vi "Finish.vi"   [LabVIEW 2015]
doc: "This VI is called just before exiting. It is expected to close I/O refnum, save collected data, etc."
uses:
  <vilib>/Rock Robotics/WPI/Utilities/WPI_GetSetVariantRefNum.vi
types:
  T1 = typedef "WPI_MotorControlDeviceRef.ctl" = cluster{"DeviceStatus":errorcluster, "Type":T2, "PWM":cluster{"PWM Channel":T3, "DeadBand":T4}, "CAN":cluster{"Device Number":u8, "Control Mode":T5, "Semaphore":T6, "Max Vout":dbl, "TalonSRX Control Mode":T7}, "Invert":bool}
  T2 = typedef "WPI_MotorControlType.ctl" = enum16{"PWM", "CAN", "CANTalonSRX"}
  T3 = typedef "FPGA_DIOPWMChannel.ctl" = enum8{"PWM 0", "PWM 1", "PWM 2", "PWM 3", "PWM 4", "PWM 5", "PWM 6", "PWM 7", "PWM 8", "PWM 9", "PWM MXP 0", "PWM MXP 1", "PWM MXP 2", "PWM MXP 3", "PWM MXP 4", "PWM MXP 5", "PWM MXP 6", "PWM MXP 7", "PWM MXP 8", "PWM MXP 9", "Invalid"}
  T4 = typedef "WPI_PWMDeadband.ctl" = cluster{"Name":string, "maxPositivePwm":i32, "minPositivePwm":i32, "centerPwm":i32, "maxNegativePwm":i32, "minNegativePwm":i32, "angularRange":u16}
  T5 = typedef "WPI_CANJaguar_ControlMode.ctl" = enum8{"Percent VBus", "Current", "Speed", "Position", "Voltage"}
  T6 = typedef "Semaphore RefNum" = refnum<k1>
  T7 = typedef "WPI_CANTalonSRX_APIControlMode.ctl" = enum8{"Percent VBus", "Speed", "Position", "Slave", "Unchanged / Invalid", "Voltage Compensation", "Current", "Motion Profile"}
  T8 = typedef "WPI_SwitchDevRef.ctl" = cluster{"DevStatus":errorcluster, "DIO Channel":T9, "CntIndex":T10, "Normally Closed":bool}
  T9 = typedef "FPGA_DIOChannel.ctl" = enum8{"DIO 0", "DIO 1", "DIO 2", "DIO 3", "DIO 4", "DIO 5", "DIO 6", "DIO 7", "DIO 8", "DIO 9", "DIO MXP 0", "DIO MXP 1", "DIO MXP 2", "DIO MXP 3", "DIO MXP 4", "DIO MXP 5", "DIO MXP 6", "DIO MXP 7", "DIO MXP 8", "DIO MXP 9", "DIO MXP 10", "DIO MXP 11", "DIO MXP 12", "DIO MXP 13", "DIO MXP 14", "DIO MXP 15", "Invalid"}
  T10 = typedef "FPGA_CounterCtrSystemIndex.ctl" = enum8{"Ctr 0", "Ctr 1", "Ctr 2", "Ctr 3", "Ctr 4", "Ctr 5", "Ctr 6", "Ctr 7", "Invalid"}
  T11 = typedef "WPI_JoystickDevRef.ctl" = cluster{"Device":T12}
  T12 = typedef "WPI_JoystickDeviceEnum.ctl" = enum16{"USB 0", "USB 1", "USB 2", "USB 3", "USB 4", "USB 5"}
  T13 = typedef "WPI_SolenoidDevRef.ctl" = cluster{"DevStatus":errorcluster, "Pneumatics Control Module":u8, "Forward Solenoid Channel":T14, "Reverse Solenoid Channel":T14}
  T14 = typedef "WPI_SolenoidChannel.ctl" = enum8{"Solenoid 0", "Solenoid 1", "Solenoid 2", "Solenoid 3", "Solenoid 4", "Solenoid 5", "Solenoid 6", "Solenoid 7", "Invalid"}
  T15 = typedef "WPI_RelayDevRef.ctl" = cluster{"DevStatus":errorcluster, "Relay Channel":T16, "Relay Direction":T17}
  T16 = typedef "FPGA_DIORelayChannel.ctl" = enum8{"Relay 0", "Relay 1", "Relay 2", "Relay 3", "Invalid"}
  T17 = typedef "WPI_RelayDirection.ctl" = enum16{"Both directions", "Forward only", "Reverse only"}
  T18 = typedef "WPI_CompressorDevRef.ctl" = cluster{"DevStatus":errorcluster, "Pneumatics Control Module":u8}
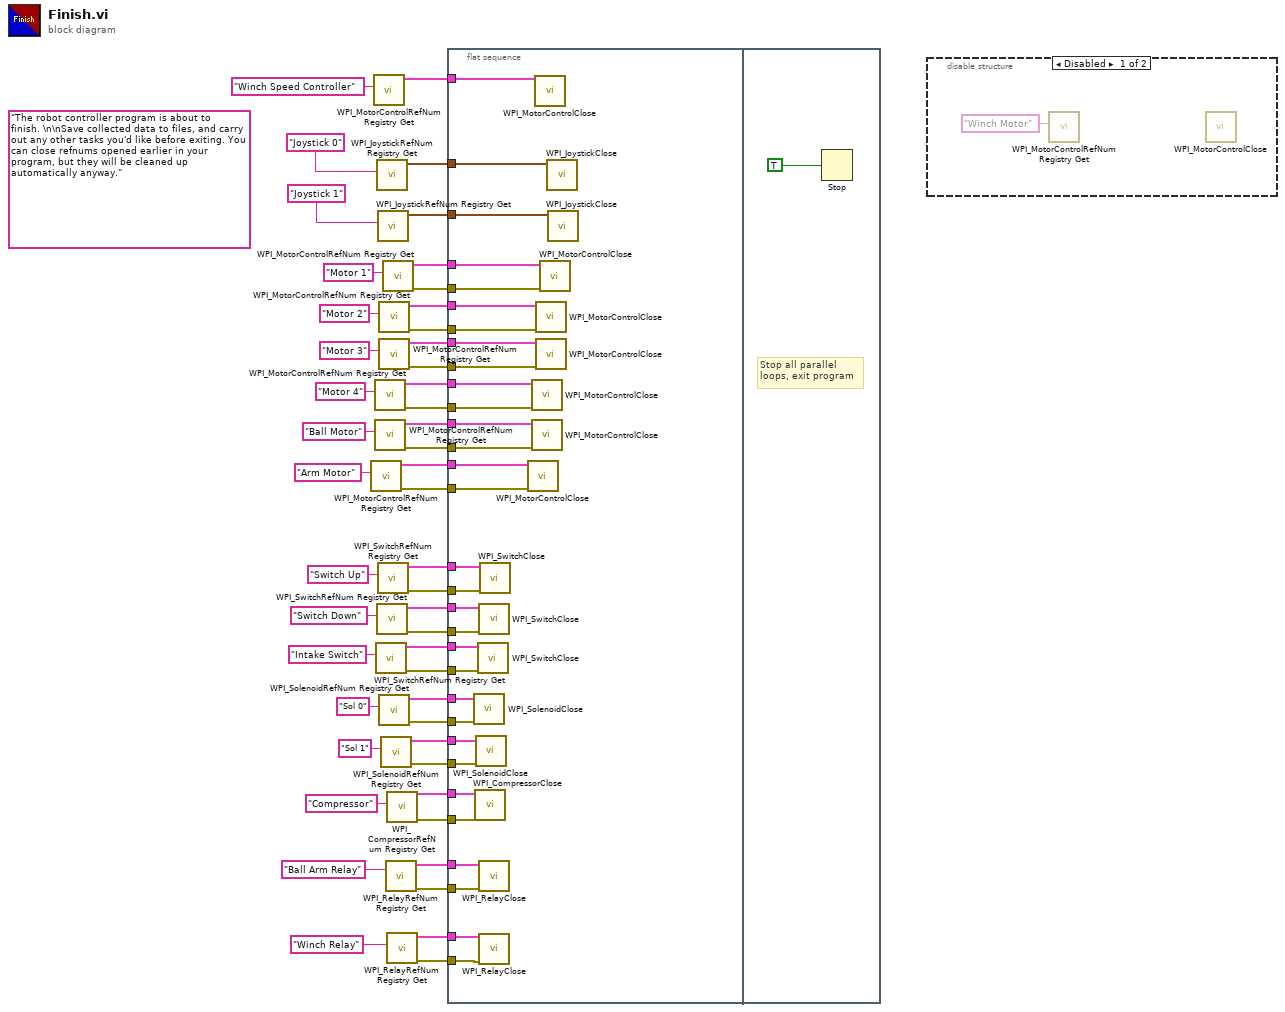
[diagram p0: block diagram]
diagram:
  (unwired) "The robot controller program is about to finish. \n\nSave collected data to files, and carry out any other tasks you'd like before exiting. You can close refnums opened earlier in your program, but they will be cleaned up automatically anyway."
  n1 = call <vilib>:"WPI_MotorControlRefNum Registry Get.vi"("refnum name"="Arm Motor") -> ("error out"=w28:errorcluster, "MotorControlDevRef"=w27:T1)  [unwired: 9 in]
  n2 = call <vilib>:"WPI_MotorControlRefNum Registry Get.vi"("refnum name"="Winch Speed Controller") -> ("MotorControlDevRef"=w2:T1)  [unwired: 9 in, 1 out]
  n3 = call <vilib>:"WPI_MotorControlRefNum Registry Get.vi"("refnum name"="Motor 4") -> ("error out"=w37:errorcluster, "MotorControlDevRef"=w38:T1)  [unwired: 9 in]
  n4 = call <vilib>:"WPI_MotorControlRefNum Registry Get.vi"("refnum name"="Ball Motor") -> ("error out"=w31:errorcluster, "MotorControlDevRef"=w32:T1)  [unwired: 9 in]
  n5 = call <vilib>:"WPI_SwitchRefNum Registry Get.vi"("refnum name"="Intake Switch") -> ("error out"=w19:errorcluster, "SwitchDevRef"=w20:T8)  [unwired: 9 in]
  n6 = call <vilib>:"WPI_JoystickRefNum Registry Get.vi"("refnum name"="Joystick 0") -> ("JoystickDevRef"=w47:T11)  [unwired: 1 in, 9 out]
  n7 = call <vilib>:"WPI_SwitchRefNum Registry Get.vi"("refnum name"="Switch Down") -> ("error out"=w22:errorcluster, "SwitchDevRef"=w21:T8)  [unwired: 9 in]
  n8 = call <vilib>:"WPI_JoystickRefNum Registry Get.vi"("refnum name"="Joystick 1") -> ("JoystickDevRef"=w46:T11)  [unwired: 1 in, 9 out]
  n9 = call <vilib>:"WPI_SwitchRefNum Registry Get.vi"("refnum name"="Switch Up") -> ("error out"=w25:errorcluster, "SwitchDevRef"=w26:T8)  [unwired: 9 in]
  n10 = call <vilib>:"WPI_MotorControlRefNum Registry Get.vi"("refnum name"="Motor 2") -> ("error out"=w40:errorcluster, "MotorControlDevRef"=w39:T1)  [unwired: 9 in]
  n11 = call <vilib>:"WPI_MotorControlRefNum Registry Get.vi"("refnum name"="Motor 3") -> ("error out"=w34:errorcluster, "MotorControlDevRef"=w33:T1)  [unwired: 9 in]
  n12 = call <vilib>:"WPI_SolenoidRefNum Registry Get.vi"("refnum name"="Sol 0") -> ("error out"=w16:errorcluster, "SolenoidDevRef"=w17:T13)  [unwired: 9 in]
  n13 = call <vilib>:"WPI_SolenoidRefNum Registry Get.vi"("refnum name"="Sol 1") -> ("error out"=w13:errorcluster, "SolenoidDevRef"=w12:T13)  [unwired: 9 in]
  n14 = call <vilib>:"WPI_MotorControlRefNum Registry Get.vi"("refnum name"="Motor 1") -> ("error out"=w43:errorcluster, "MotorControlDevRef"=w44:T1)  [unwired: 9 in]
  n15 = call <vilib>:"WPI_RelayRefNum Registry Get.vi"("refnum name"="Ball Arm Relay") -> ("error out"=w5:errorcluster, "RelayDevRef"=w7:T15)  [unwired: 9 in]
  n16 = call <vilib>:"WPI_CompressorRefNum Registry Get.vi"("refnum name"="Compressor") -> ("error out"=w10:errorcluster, "CompressorDevRef"=w11:T18)  [unwired: 9 in]
  n17 = call <vilib>:"WPI_RelayRefNum Registry Get.vi"("refnum name"="Winch Relay") -> ("error out"=w6:errorcluster, "RelayDevRef"=w8:T15)  [unwired: 9 in]
  n18 = flat-sequence {
    tunnel: w47 -> [w79]
    tunnel: w46 -> [w78]
    tunnel: w44 -> [w77]
    tunnel: w43 -> [w76]
    tunnel: w39 -> [w74]
    tunnel: w40 -> [w75]
    tunnel: w33 -> [w70]
    tunnel: w34 -> [w71]
    tunnel: w38 -> [w73]
    tunnel: w37 -> [w72]
    tunnel: w32 -> [w69]
    tunnel: w31 -> [w68]
    tunnel: w27 -> [w66]
    tunnel: w28 -> [w67]
    tunnel: w26 -> [w65]
    tunnel: w25 -> [w64]
    tunnel: w21 -> [w62]
    tunnel: w22 -> [w63]
    tunnel: w20 -> [w61]
    tunnel: w19 -> [w60]
    tunnel: w17 -> [w59]
    tunnel: w16 -> [w58]
    tunnel: w12 -> [w56]
    tunnel: w13 -> [w57]
    tunnel: w11 -> [w55]
    tunnel: w10 -> [w54]
    tunnel: w8 -> [w53]
    tunnel: w7 -> [w52]
    tunnel: w6 -> [w51]
    tunnel: w5 -> [w50]
    tunnel: w2 -> [w49]
    frame #0 {
      n19 = call <vilib>:"WPI_SolenoidClose.vi"("error in (no error)"=w58, "SolenoidDevRef"=w59) -> ()  [unwired: 9 in, 1 out]
      n20 = call <vilib>:"WPI_CompressorClose.vi"("error in (no error)"=w54, "CompressorDevRef"=w55) -> ()  [unwired: 9 in, 1 out]
      n21 = call <vilib>:"WPI_SolenoidClose.vi"("error in (no error)"=w57, "SolenoidDevRef"=w56) -> ()  [unwired: 9 in, 1 out]
      n22 = call <vilib>:"WPI_SwitchClose.vi"("error in (no error)"=w60, "SwitchDevRef"=w61) -> ()  [unwired: 9 in, 1 out]
      n23 = call <vilib>:"WPI_SwitchClose.vi"("error in (no error)"=w63, "SwitchDevRef"=w62) -> ()  [unwired: 9 in, 1 out]
      n24 = call <vilib>:"WPI_RelayClose.vi"("error in (no error)"=w50, "RelayDevRef"=w52) -> ()  [unwired: 9 in, 1 out]
      n25 = call <vilib>:"WPI_RelayClose.vi"("error in (no error)"=w51, "RelayDevRef"=w53) -> ()  [unwired: 9 in, 1 out]
      n26 = call <vilib>:"WPI_SwitchClose.vi"("error in (no error)"=w64, "SwitchDevRef"=w65) -> ()  [unwired: 9 in, 1 out]
      n27 = call <vilib>:"WPI_MotorControlClose.vi"("error in (no error)"=w67, "MotorControlDevRef"=w66) -> ()  [unwired: 9 in, 1 out]
      n28 = call <vilib>:"WPI_MotorControlClose.vi"("error in (no error)"=w72, "MotorControlDevRef"=w73) -> ()  [unwired: 9 in, 1 out]
      n29 = call <vilib>:"WPI_MotorControlClose.vi"("error in (no error)"=w68, "MotorControlDevRef"=w69) -> ()  [unwired: 9 in, 1 out]
      n30 = call <vilib>:"WPI_MotorControlClose.vi"("MotorControlDevRef"=w49) -> ()  [unwired: 10 in, 1 out]
      n31 = call <vilib>:"WPI_MotorControlClose.vi"("error in (no error)"=w75, "MotorControlDevRef"=w74) -> ()  [unwired: 9 in, 1 out]
      n32 = call <vilib>:"WPI_MotorControlClose.vi"("error in (no error)"=w71, "MotorControlDevRef"=w70) -> ()  [unwired: 9 in, 1 out]
      n33 = call <vilib>:"WPI_MotorControlClose.vi"("error in (no error)"=w76, "MotorControlDevRef"=w77) -> ()  [unwired: 9 in, 1 out]
      n34 = call <vilib>:"WPI_JoystickClose.vi"("JoystickDevRef"=w79) -> ()  [unwired: 11 out]
      n35 = call <vilib>:"WPI_JoystickClose.vi"("JoystickDevRef"=w78) -> ()  [unwired: 11 out]
    }
    frame #1 {
      # "Stop all parallel\nloops, exit program"
      n36 = Stop(stop? (T)=TRUE ("Quit")) -> ()
    }
  }
  n37 = disable-structure shown="Disabled" {
    frame Disabled {
      n38 = call <vilib>:"WPI_MotorControlRefNum Registry Get.vi"("refnum name"="Winch Motor") -> ("error out"=w82:errorcluster, "MotorControlDevRef"=w81:T1)  [unwired: 9 in]
      n39 = call <vilib>:"WPI_MotorControlClose.vi"() -> ("error in (no error)"=w85:errorcluster, "MotorControlDevRef"=w84:T1)  [unwired: 9 in, 1 out]
    }
    frame Enabled {
    }
  }
